vi "parseErrorCheck_roslv.vi"(1 "type":string, 2 "error in":errorcluster, 3 "msg read":string) -> (0 "error out":errorcluster)   [LabVIEW 2014]
doc: "Parses a message into an error check"
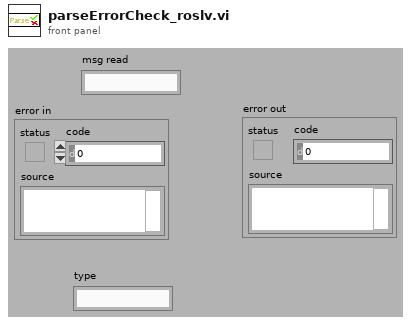
[diagram p1: front panel]
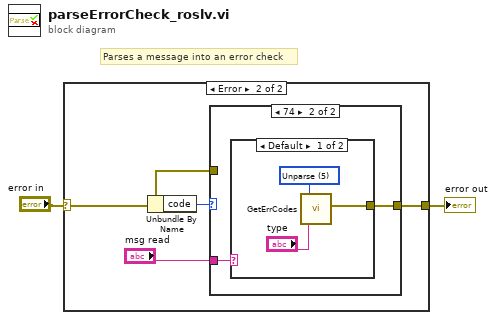
[diagram p0: block diagram]
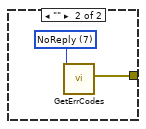
[diagram p4: hidden frame]
diagram:
  # "Parses a message into an error check"
  n1 = case shown="Error" "error in" {
    selector: "error in" -> [w3 w5]
    tunnel: [w3 w7] -> w1
    frame No Error {
    }
    frame Error {
      n2 = Unbundle By Name(w5) -> ("code"=w6:i32)
      n3 = case shown="74" w6 {
        tunnel: [w8 w10] -> w7
        tunnel: w5 -> [w8 _]
        tunnel: "msg read" -> [_ w9]
        frame Default {
        }
        frame 74 {
          n4 = case shown="Default" w9 {
            tunnel: [w12 w15] -> w10
            frame Default {
              w13 = u16 5 items=["TopicReadTimeout", "Read=SS", "GetQueueErr", "NoMaster", "Write=PS", "Unparse"] ("Error")
              n5 = call "GetErrCodes.vi"("Added Text"="type", "Error"=w13) -> ("Error"=w12:errorcluster)
            }
            frame "" {
              w14 = u16 7 items=["TopicReadTimeout", "Read=SS", "GetQueueErr", "NoMaster", "Write=PS", "Unparse", "ServiceReply", "NoReply"] ("Error")
              n6 = call "GetErrCodes.vi"("Error"=w14) -> ("Error"=w15:errorcluster)  [unwired: 1 in]
            }
          }
        }
      }
    }
  }
  "error out" <- w1
